vi "Untitled 1.vi"() -> ()   [LabVIEW 2016]
uses:
  <vilib>/userdefined/High Color/IMAQdx.ctl
  <vilib>/vision/Classification.llb/IMAQ Classifier Session.ctl
  <vilib>/vision/driver/NI_Vision_Acquisition_Software.lvlib
  <resource>/objmgr/imaqdx.rc
panel:
  out "color":string
  out "error out 2":errorcluster
  out "Classes (Color Classification 1)":string[](array[string])
  out "Classifier Session (Color Classification 1)":T1
  out "source":T2(plugin-control)
  out "processed":T2(plugin-control)
  in  "error in (no error)":errorcluster
  in  "video mode":u32
  in  "webcam":T3="cam0"
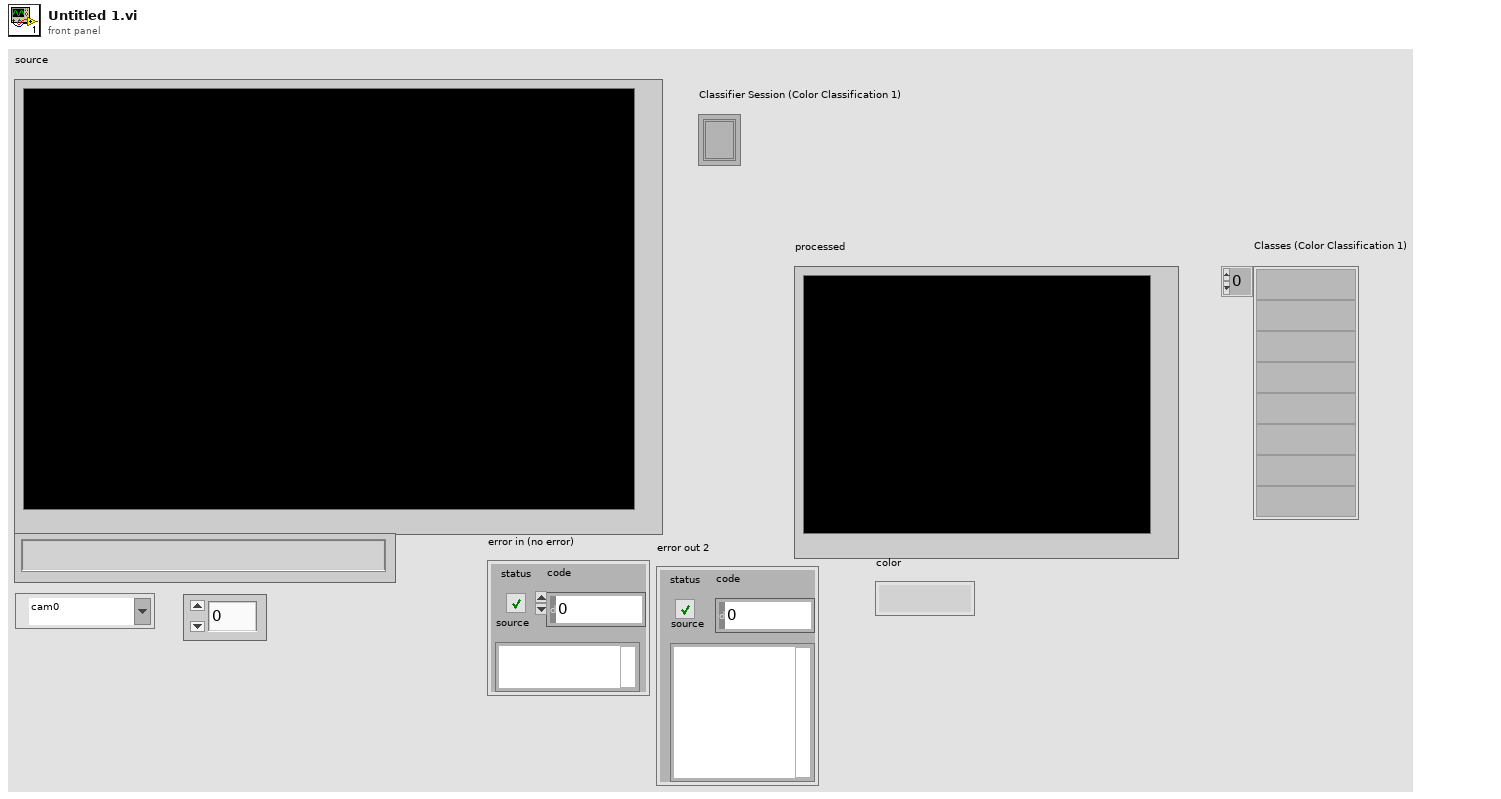
[diagram p1: front panel]
types:
  T1 = typedef "IMAQ Classifier Session.ctl" = refnum<k1>
  T2 = typedef "IMAQ Image.ctl" = refnum<image>
  T3 = typedef "IMAQdx.ctl" = refnum<k21>
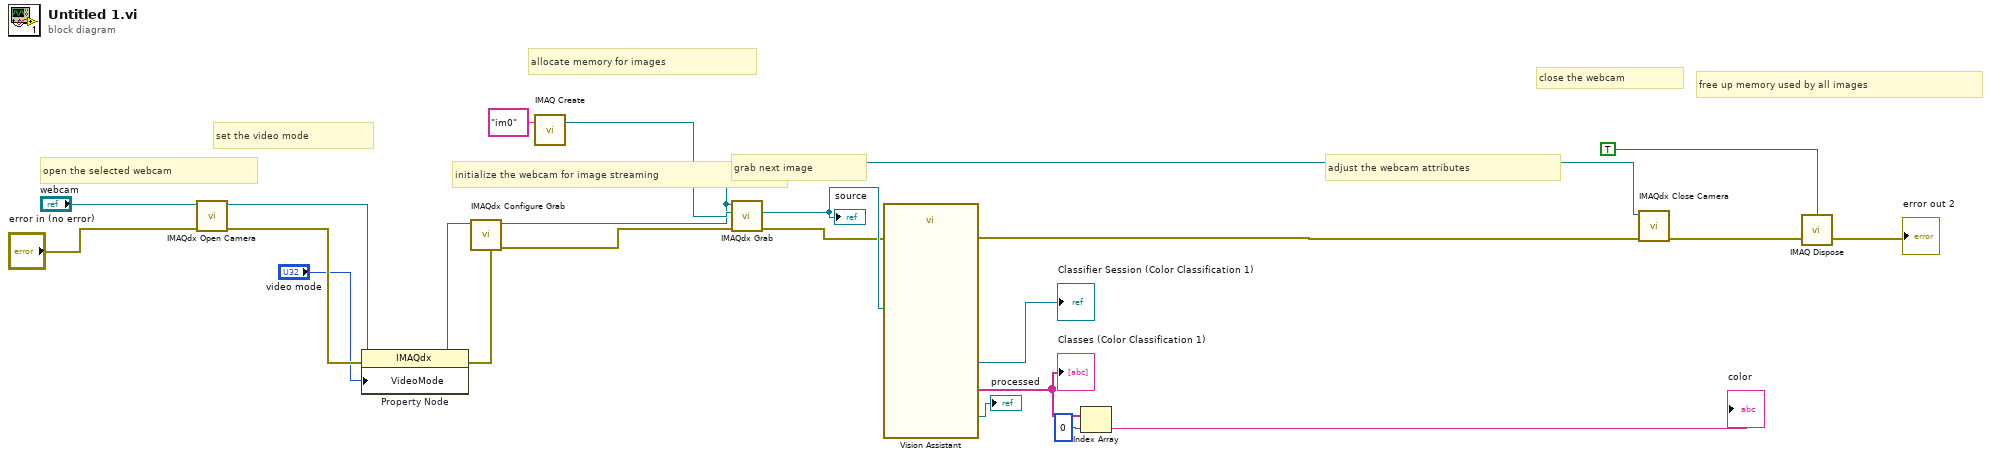
[diagram p0: block diagram]
diagram:
  # "adjust the webcam attributes"
  # "grab next image"
  # "close the webcam"
  # "open the selected webcam"
  # "set the video mode"
  # "allocate memory for images"
  # "initialize the webcam for image streaming"
  # "free up memory used by all images"
  n1 = call <vilib>:"IMAQdx Open Camera.vi"("error in"="error in (no error)", "Session In"="webcam") -> ("error out"=w15:errorcluster, "Session Out"=w14:T3)  [unwired: 1 in, 7 out]
  n2 = property on="Property Node" class="IMAQdx"(reference=w14, error in=w15, "VideoMode"="video mode") -> (reference out=w11:T3, error out=w12:errorcluster)
  n3 = call <vilib>:"IMAQdx Configure Grab.vi"("error in"=w12, "Session In"=w11) -> ("error out"=w19:errorcluster, "Session Out"=w16:T3)  [unwired: 8 in]
  n4 = call "IMAQ Create"("Image Name"="im0") -> ("New Image"=w20:T2)  [unwired: 3 in, 2 out]
  n5 = call <vilib>:"IMAQdx Grab.vi"("error in"=w19, "Image In"=w20, "Session In"=w16) -> ("error out"=w8:errorcluster, "Image Out"=w9:T2)  [unwired: 5 in, 2 out]
  "source" <- w9
  n6 = call "Vision Assistant"("Image In"=w9, "error in"=w8) -> ("Image Out"=→"processed":T2, "Classifier Session (Color Classification 1)"=→"Classifier Session (Color Classification 1)":T1, "Classes (Color Classification 1)"=w4:string[], "error out"=w1:errorcluster)  [unwired: 22 in]
  "Classes (Color Classification 1)" <- w4
  n7 = Index Array(array=w4, index=0) -> (element=→"color":string)
  n8 = call <vilib>:"IMAQdx Close Camera.vi"("error in"=w1, "Session In"=w16) -> ("error out"=w17:errorcluster)  [unwired: 9 out]
  n9 = call "IMAQ Dispose"("All Images? (No)"=TRUE, "error in (no error)"=w17) -> ("error out"=→"error out 2":errorcluster)  [unwired: 4 in]
